vi "Acquire_org.vi"(7 "Signal Type":T1, 8 "error in (no error)":errorcluster, 11 "HW ID in":string) -> (0 "error out":errorcluster, 2 "Graph Data":waveform(dbl)[](array[waveform]), 3 "HW ID out":string)   [LabVIEW 2019]
doc: "Perform the acquisition. Replace the contents of this diagram with calls to acquisition hardware.\n_____\nBased on DQMH Project Template 6.0.0.91."
uses:
  CML Shared/Signal Type--enum.ctl
  <vilib>/ULx/Read.llb/ULx Read (Analog 1D DBL NChan 1Samp).vi
  <vilib>/ULx/Create Channel.llb/ULx Create Channel (AI-Temperature).vi
  CML Shared/CML Shared.lvlib
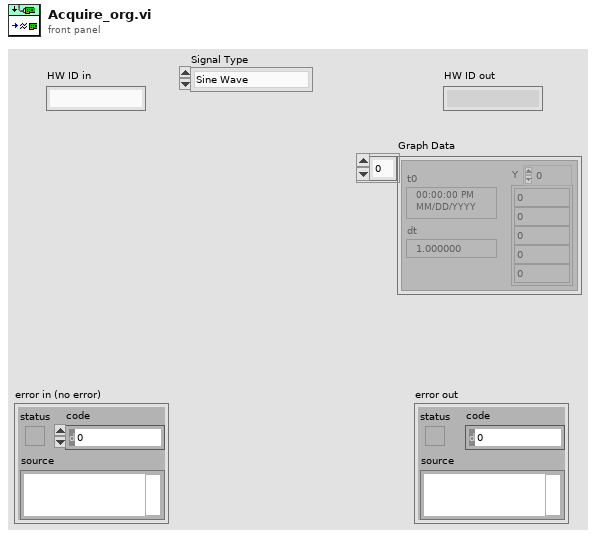
[diagram p1: front panel]
types:
  T1 = typedef "CML Shared.lvlib/Signal Type--enum.ctl" = enum16{"Sine Wave", "Square with Noise"}
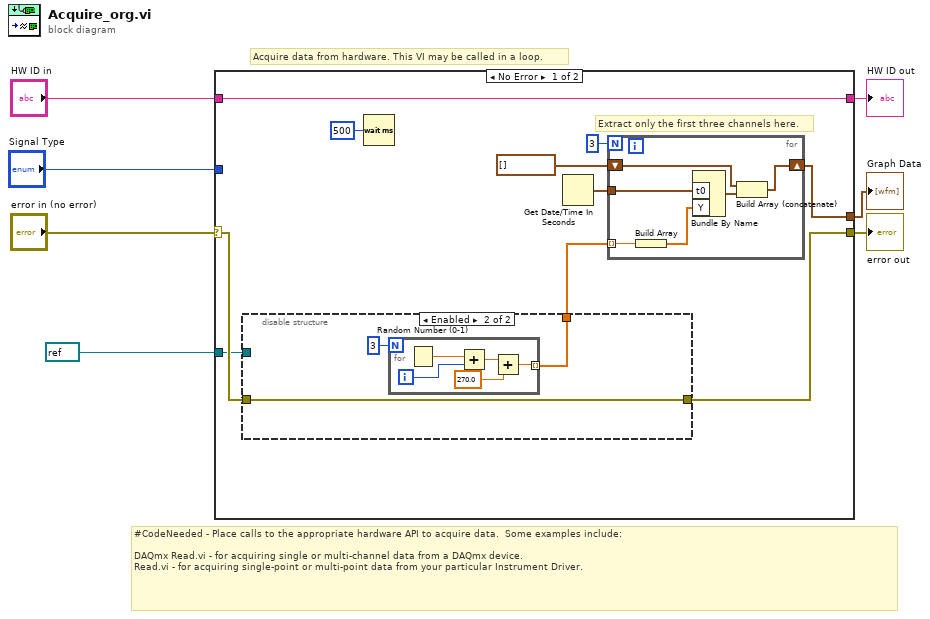
[diagram p0: block diagram]
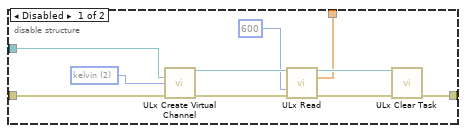
[diagram p2: hidden frame]
diagram:
  # "Acquire data from hardware. This VI may be called in a loop."
  # "#CodeNeeded - Place calls to the appropriate hardware API to acquire data.  Some examples include:\n\nDAQmx Read.vi - for acquiring single or multi-channel data from a DAQmx device.\nRead.vi - for acquiring single-point or multi-point data from your particular Instrument Driver."
  n1 = case shown="No Error" "error in (no error)" {
    selector: "error in (no error)" -> [w10 w42]
    tunnel: [w11 w42] -> w6
    tunnel: "HW ID in" -> [w17 w43]
    tunnel: [w17 w43] -> w4
    tunnel: "Signal Type" -> [_ _]
    tunnel: [w13 _] -> w2
    tunnel: refnum<k21> refnum ("Refnum in") -> [w9 _]
    frame No Error {
      # "Extract only the first three channels here."
      n2 = disable-structure shown="Enabled" {
        disable-tunnel: [w22 w30] -> w11
        disable-tunnel: w10 -> [w21 w30]
        disable-tunnel: w9 -> [w20 _]
        disable-tunnel: [w18 w28] -> w12
        frame Disabled {
          w19 = 2 items=["degC", "degF", "kelvin", "raw"] ("units")
          n3 = call-poly <vilib>:"ULx Create Virtual Channel.vi"("physical channels"=w20, "units"=w19, "error in"=w21) -> ("task out"=w26:refnum<k24>, "error out"=w27:errorcluster)  [unwired: 11 in]
          n4 = call-poly <vilib>:"ULx Read.vi"("task in"=w26, "timeout"=600, "error in"=w27) -> ("task out"=w25:refnum<k24>, "data"=w18:dbl[], "error out"=w24:errorcluster)  [unwired: 10 in]
          n5 = call <vilib>:"ULx Clear Task.vi"("task in"=w25, "error in"=w24) -> ("error out"=w22:errorcluster)  [unwired: 13 in]
        }
        frame Enabled {
          n6 = for {
            N: 3 -> [_]
            tunnel: [w33] -> w28 mode=indexing
            i -> [w34]
            n7 = Random Number (0-1)() -> (number: 0 to 1=w35:dbl)
            n8 = Add(x=w35, y=w34) -> (x+y=w32:dbl)
            n9 = Add(x=w32, y=270.0) -> (x+y=w33:dbl)
          }
        }
      }
      n10 = Wait (ms)(milliseconds to wait=u32 500) -> ()  [unwired: 1 out]
      n11 = Get Date/Time In Seconds() -> (seconds since 1Jan1904=w16:timestamp)
      n12 = for {
        N: 3 -> [_]
        tunnel: w16 -> [w41]
        tunnel: w12 -> [w40] mode=indexing
        shift-right: [w38] -> w13
        shift-left: waveform(dbl)[] [] -> [w37]
        n13 = Build Array(w40) -> (w39:dbl[])
        n14 = Bundle By Name("t0"=w41, "Y"=w39) -> (w36:waveform(dbl))  [unwired: 1 in]
        n15 = Build Array (concatenate)(w37, w36) -> (w38:waveform(dbl)[])
      }
    }
    frame Error {
    }
  }
  "HW ID out" <- w4
  "error out" <- w6
  "Graph Data" <- w2
